vi "Send WernerReadback.vi"(7 "Message Priority (Normal)":T1=enum."Normal", 8 "error in (no error)":errorcluster, 9 "Value":u32, 10 "URL":string, 11 "Message Enqueuer":refnum<class "Message Enqueuer.lvclass">) -> (0 "error out":errorcluster, 3 "Message Enqueuer out":refnum<class "Message Enqueuer.lvclass">)   [LabVIEW 2015, in "CS++IEFWerner.lvlib" / "Update_Readback Msg.lvclass"]
doc: "Sends the <B>CS++IEFWerner.lvlib:WernerReadback Msg.lvclass</B> message.\n\n<B>CS++IEFWerner.lvlib:CS++IEFWerner.lvclass:WernerReadback.vi</B> Description:\n\nThis VI gets the infos from the Status SV of the IEF motor controller, makes some calculations and updates the important SVs."
uses:
  Update_Readback Msg.lvclass
  <vilib>/ActorFramework/Message Enqueuer/Message Enqueuer.lvclass
  <vilib>/ActorFramework/Message Enqueuer/Message Priority.ctl
  Update_Readback Msg.lvclass/Update_Readback Msg.ctl
  <vilib>/ActorFramework/Message Enqueuer/Message Enqueuer.lvclass/Message Enqueuer.ctl
  <vilib>/ActorFramework/Message Priority Queue/Priority Enqueue.vi
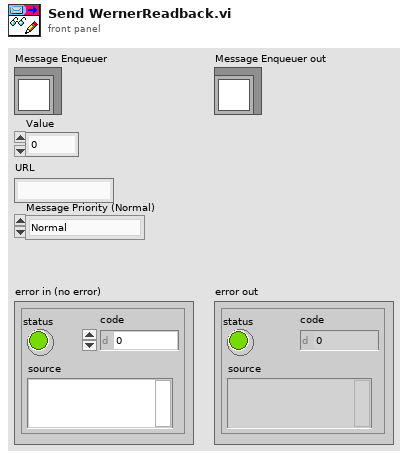
[diagram p1: front panel]
types:
  T1 = typedef "Actor Framework.lvlib/Message Enqueuer.lvclass/Message Priority.ctl" = enum16{"Low", "Normal", "High"}
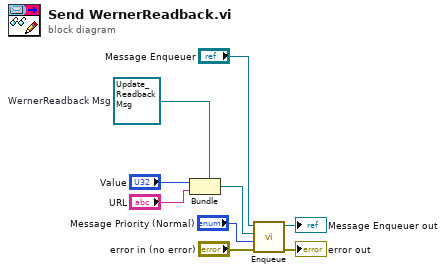
[diagram p0: block diagram]
diagram:
  w3 = refnum<class "Update_Readback Msg.lvclass"> refnum  # WernerReadback Msg
  n1 = Bundle(cluster=w3, "Value", "URL") -> (w6:refnum<class "Update_Readback Msg.lvclass">)
  n2 = call <vilib>:"Enqueue.vi"("error in (no error)"="error in (no error)", "Message Priority (Normal)"="Message Priority (Normal)", "Message"=w6, "Message Enqueuer in"="Message Enqueuer") -> ("error out"=→"error out":errorcluster, "Message Enqueuer out"=→"Message Enqueuer out":refnum<class "Message Enqueuer.lvclass">)  [unwired: 6 in]
